vi "Get_Intersections.vi"(6 "color":u32(colorbox)=65316, 8 "Draw?":bool=TRUE, 10 "Edge Points":cluster{dbl, dbl}[][](array[cluster]), 11 "picture in":picture) -> (2 "All Points":cluster{"x":dbl, "y":dbl}[][](array[cluster]), 3 "picture out":picture)   [LabVIEW 2022 SP3]
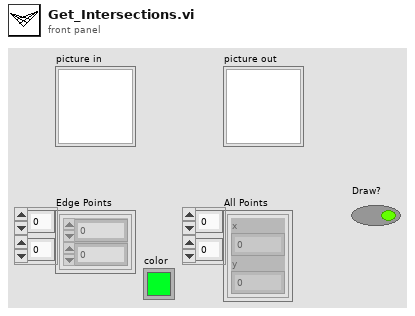
[diagram p1: front panel]
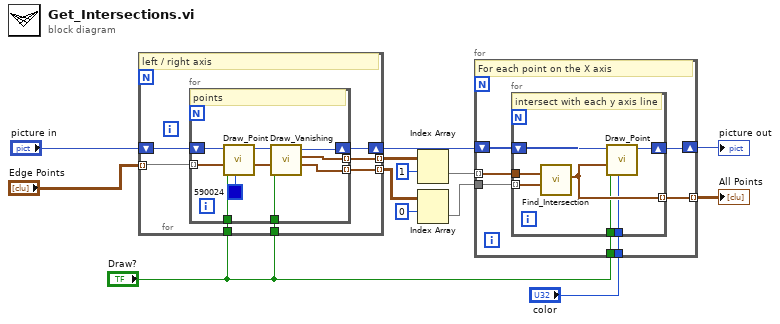
[diagram p0: block diagram]
diagram:
  n1 = for {
    shift-right: [w20] -> w5
    shift-left: "picture in" -> [w19]
    tunnel: "Edge Points" -> [w18] mode=indexing
    tunnel: [w16] -> w6 mode=indexing
    tunnel: [w17] -> w10 mode=indexing
    tunnel: "Draw?" -> [w15]
    tunnel: "Draw?" -> [w14]
    # "left / right axis"
    n2 = for {
      tunnel: w18 -> [w25] mode=indexing
      shift-right: [w29] -> w20
      shift-left: w19 -> [w28]
      tunnel: [w24] -> w16 mode=indexing
      tunnel: [w23] -> w17 mode=indexing
      tunnel: w15 -> [w22]
      tunnel: w14 -> [w21]
      # "points"
      n3 = call "Draw_Point.vi"("color"=u32 590024, "Draw?"=w22, "point"=w25, "picture in"=w28) -> ("new picture"=w26:picture)  [unwired: 7 in]
      n4 = call "Draw_Vanishing.vi"("Draw?"=w21, "point"=w25, "picture in"=w26) -> ("right_line"=w23:cluster{"slope":dbl, "b":dbl, "theta":dbl}, "left_line"=w24:cluster{"slope":dbl, "b":dbl, "theta":dbl}, "picture out"=w29:picture)  [unwired: 6 in]
    }
  }
  n5 = Index Array(array=w6, index (row)=1) -> (element=w8:cluster{"slope":dbl, "b":dbl, "theta":dbl}[])  [unwired: 1 in]
  n6 = Index Array(array=w10, index (row)=0) -> (element=w11:cluster{"slope":dbl, "b":dbl, "theta":dbl}[])  [unwired: 1 in]
  n7 = for {
    tunnel: w8 -> [w36] mode=indexing
    shift-right: [w34] -> w13
    shift-left: w5 -> [w35]
    tunnel: w11 -> [w33]
    tunnel: [w32] -> w12 mode=indexing
    tunnel: "color" -> [w31]
    tunnel: "Draw?" -> [w30]
    # "For each point on the X axis"
    n8 = for {
      tunnel: w36 -> [w41]
      shift-right: [w42] -> w34
      shift-left: w35 -> [w43]
      tunnel: w33 -> [w40] mode=indexing
      tunnel: [w39] -> w32 mode=indexing
      tunnel: w31 -> [w38]
      tunnel: w30 -> [w37]
      # "intersect with each y axis line"
      n9 = call "Find_Intersection.vi"("line 2"=w40, "line 1"=w41) -> ("Intersection"=w39:cluster{"x":dbl, "y":dbl})  [unwired: 9 in]
      n10 = call "Draw_Point.vi"("color"=w38, "Draw?"=w37, "point"=w39, "picture in"=w43) -> ("new picture"=w42:picture)  [unwired: 7 in]
    }
  }
  "picture out" <- w13
  "All Points" <- w12
